vi "Basics - Loops, Case Structure, StateMachine.vi"   [LabVIEW 2023]
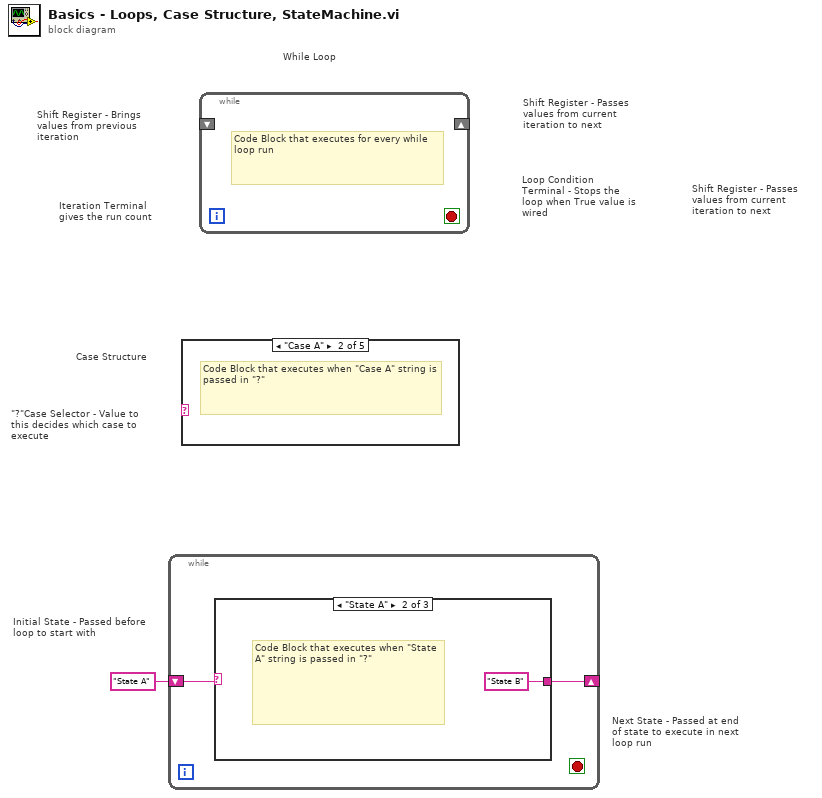
[diagram p0: block diagram]
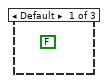
[diagram p6: hidden frame]
diagram:
  # "Next State - Passed at end of state to execute in next loop run"
  # "Initial State - Passed before loop to start with"
  # "\"?\"Case Selector - Value to this decides which case to execute"
  # "Shift Register - Passes values from current iteration to next"
  # "Case Structure"
  # "While Loop"
  # "Shift Register - Brings values from previous iteration"
  # "Shift Register - Passes values from current iteration to next"
  # "Loop Condition Terminal - Stops the loop when True value is wired"
  # "Iteration Terminal  gives the run count"
  n1 = while {
    shift-right: [w2] -> _
    shift-left: "State A" ("Initial State") -> [w3]
    stop <- _ stop-if-true
    n2 = case shown="\"State A\"" w3 {
      selector: w3 -> [_ _ w5]
      tunnel: [_ "State B" ("Next State") w5] -> w2
      frame Default {
        (unwired) FALSE ("Data Received?")
      }
      frame "State A" {
        # "Code Block that executes when \"State A\" string is passed in \"?\""
      }
      frame "XYZ" {
      }
    }
  }
  n3 = case "Executes code based on Model Name" shown="\"Case A\"" {
    selector: _ -> [_ _ _ _ _]
    frame Default {
    }
    frame "Case A" {
      # "Code Block that executes when \"Case A\" string is passed in \"?\""
    }
    frame "Case B" {
    }
    frame "Case C" {
    }
    frame "Case D" {
    }
  }
  n4 = while {
    shift-right: _ -> [_]
    shift-left: _ -> [_]
    stop <- _ stop-if-true
    # "Code Block that executes for every while loop run"
  }
